vi "VSI Block Read Bytes.vi"(5 "IntervalTime":u32, 6 "BlockNum":u16, 7 "BlockSize":u16, 9 "SPIIndex":i32, 10 "DevIndex":i32, 11 "DevType":i32) -> (2 "function return":i32, 3 "pReadData":u8[](array[numeric]))   [LabVIEW 2010, in "ControlSPI.lvlib"]
doc: "int WINAPI VSI_BlockReadBytes(int DevType,int DevIndex,int SPIIndex,unsigned char *pReadData,unsigned short BlockSize,unsigned short BlockNum,unsigned int IntervalTime);"
uses:
  ControlSPI.lvlib
  ControlSPI/Ginkgo_Driver.dll
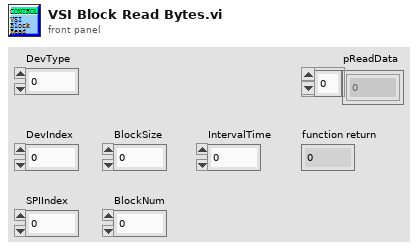
[diagram p1: front panel]
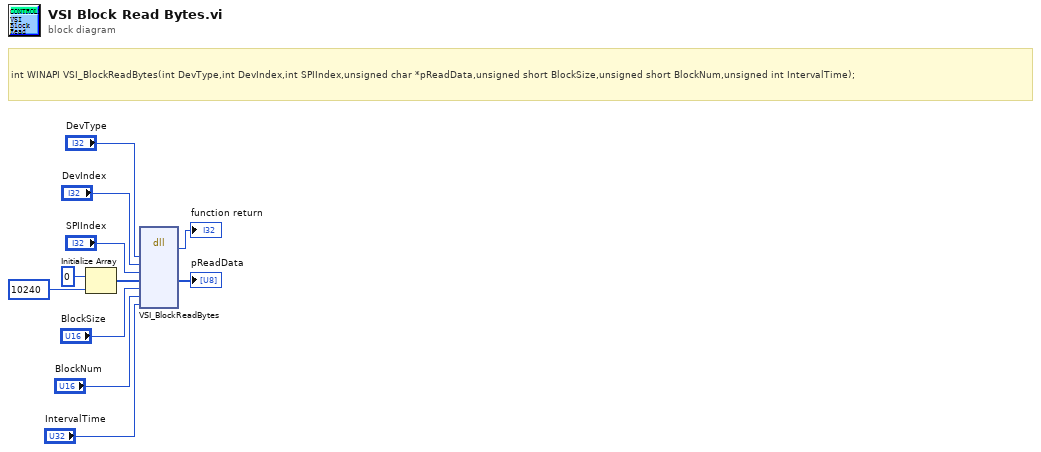
[diagram p0: block diagram]
diagram:
  # "int WINAPI VSI_BlockReadBytes(int DevType,int DevIndex,int SPIIndex,unsigned char *pReadData,unsigned short BlockSize,unsigned short BlockNum,unsigned int IntervalTime);"
  n1 = Initialize Array(u8 0 ("element"), 10240 ("dimension size")) -> (w7:u8[])
  n2 = dll-call lib="E:/Project/vt_ginkgo/truck/Ginkgo Driver/vs2010/Ginkgo_USB-I2C&SPI&CAN_API_v2.0.3.3/lib/labview_32bit/ControlSPI/Ginkgo_Driver.*" fn="VSI_BlockReadBytes"("DevType"="DevType", "DevIndex"="DevIndex", "SPIIndex"="SPIIndex", "pReadData"=w7, "BlockSize"="BlockSize", "BlockNum"="BlockNum", "IntervalTime"="IntervalTime") -> (→"function return":i32, "pReadData"=→"pReadData":u8[])  [unwired: 9 in, 2 out]
